vi "Spark MAX Unpack Faults.vi"(5 "Numeric":u16) -> (2 "Faults out":T1)   [LabVIEW 2023]
uses:
  Typedef/SPARK Faults.ctl
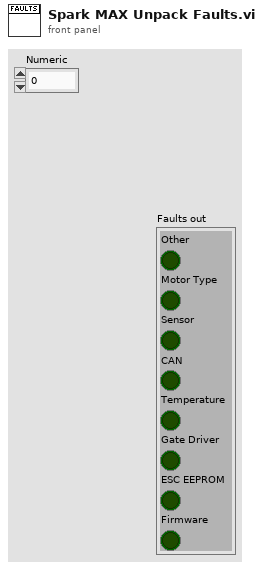
[diagram p1: front panel]
types:
  T1 = typedef "SPARK Faults.ctl" = cluster{"Other":bool, "Motor Type":bool, "Sensor":bool, "CAN":bool, "Temperature":bool, "Gate Driver":bool, "ESC EEPROM":bool, "Firmware":bool}
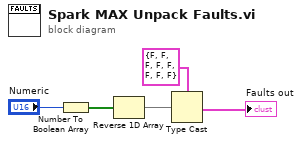
[diagram p0: block diagram]
diagram:
  n1 = Number To Boolean Array(number="Numeric") -> (Boolean array=w4:bool[])
  n2 = Reverse 1D Array(array=w4) -> (reversed array=w1:bool[])
  n3 = Type Cast(type=T1 {"Other"=FALSE, "Motor Type"=FALSE, "Sensor"=FALSE, "CAN"=FALSE, "Temperature"=FALSE, "Gate Driver"=FALSE, "ESC EEPROM"=FALSE, "Firmware"=FALSE} ("Faults out 2"), x=w1) -> (*(type *) &x=→"Faults out":T1)
